vi "fileAsynchronousClose.vi"   [LabVIEW 2017]
uses:
  globalUtilities.vi
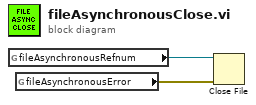
[diagram p0: block diagram]
diagram:
  n1 = global read "globalUtilities.vi" "fileAsynchronousRefnum"() -> (w2:refnum<file>)
  n2 = global read "globalUtilities.vi" "fileAsynchronousError"() -> (w1:errorcluster)
  n3 = Close File(refnum=w2, error in=w1) -> ()  [unwired: 2 out]
